vi "PCO_ForceTrigger.vi"(8 "error in (no error)":errorcluster {"code" format="%x"}, 11 "ph":u64) -> (0 "error out":errorcluster {"code" format="%x"}, 1 "wTriggered":u16(ring) items=["failed", "new image triggered"], 2 "ErrorMessage":i32 format="%x", 3 "ph out":u64)   [LabVIEW 2019, in "SDK.lvlib" / "TimingControl.lvlib"]
doc: "<b>Description:</b>\nThis function does start an exposure, if the trigger mode is either [software trigger] or [extern exposure & software trigger]. In all other trigger modes the command has no effect.\nTo accept a force trigger command the camera must be in PCO_SetRecordingState [run] and camera busy state must be [not busy] (see PCO_GetCameraBusyStatus).\n\nIf a trigger command is not accepted by the camera it is lost and will not trigger future exposures.\n• Due to response and processing times, e.g. caused by the interface and / or the operating system on the computer, the delay between command and current trigger may be several milliseconds\n• A force trigger command will be processed independent of the selected acquire mode and independent of the state of the <acq enbl> input\n• Triggers are not accumulated or buffered. A trigger will be accepted only if the camera is idle\n\n<b>Supported camera type:</b>\nAll cameras\n\n<b>Descriptor dependency:</b>\nNone"
uses:
  TimingControl.lvlib
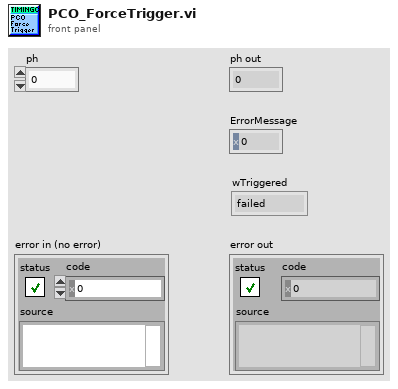
[diagram p1: front panel]
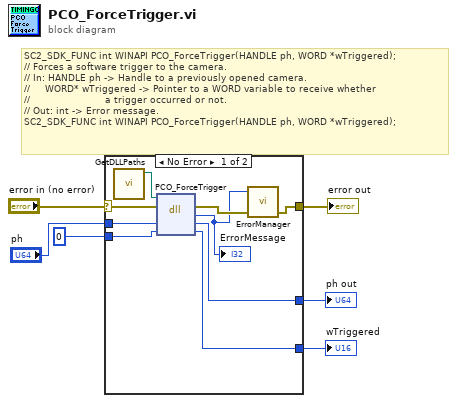
[diagram p0: block diagram]
diagram:
  # "SC2_SDK_FUNC int WINAPI PCO_ForceTrigger(HANDLE ph, WORD *wTriggered);\n// Forces a software trigger to the camera.\n// In: HANDLE ph -> Handle to a previously opened camera.\n//     WORD* wTriggered -> Pointer to a WORD variable to receive whether\n//                         a trigger occurred or not.\n// Out: int -> Error message.\nSC2_SDK_FUNC int WINAPI PCO_ForceTrigger(HANDLE ph, WORD *wTriggered);"
  n1 = case shown="No Error" "error in (no error)" {
    selector: "error in (no error)" -> [w11 w18]
    tunnel: "ph" -> [w15 w17]
    tunnel: [w14 w17] -> w5
    tunnel: u16 0 ("wTriggered") -> [w13 w16]
    tunnel: [w12 w16] -> w3
    tunnel: [w9 w18] -> w2
    frame No Error {
      n2 = call "GetDLLPaths.vi"() -> ("SC2_Cam_Path"=w7:path)  [unwired: 8 in, 3 out]
      n3 = dll-call lib="?" fn="PCO_ForceTrigger"(path in=w7, error in=w11, "ph"=w15, "wTriggered"=w13) -> (error out=w10:errorcluster, "return type"=w8:i32, "ph"=w14:u64, "wTriggered"=w12:u16)  [unwired: 1 in, 1 out]
      "ErrorMessage" <- w8
      n4 = call "ErrorManager.vi"("error in (no error)"=w10, "error code"=w8) -> ("error out"=w9:errorcluster)  [unwired: 2 in, 1 out]
    }
    frame Error {
    }
  }
  "ph out" <- w5
  "wTriggered" <- w3
  "error out" <- w2
